vi "EvenOrOdd.vi"(3 "Number":dbl) -> (1 "Even(T) or Odd(F)":bool)   [LabVIEW 2013]
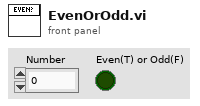
[diagram p1: front panel]
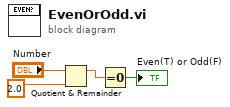
[diagram p0: block diagram]
diagram:
  n1 = Quotient & Remainder(x="Number", y=2.0) -> (x-y*floor(x/y)=w2:dbl)  [unwired: 1 out]
  n2 = Equal To 0?(x=w2) -> (x = 0?=→"Even(T) or Odd(F)":bool)
